vi "MovePilMotToRef.vi"(6 "Type de mouvement":T1 items=["Mouvement Simple"=1, "Aller vers Cote"=2], 7 "Variables d'Axes":T2={"OrdreBloc"="ni.var.psp://localhost/OPC/OPC1/esbimETH_1/module1/2AXBOC/E0_Ordre/Axe1_OrdreBloc", "Ordre UC"="ni.var.psp://localhost/OPC/OPC1/esbimETH_1/module1/2AXBOC/E0_Ordre/Axe1_OrdreUC", "CoteAAtteindre"="ni.var.psp://localhost/OPC/OPC1/esbimETH_1/module1/2AXBOC/E1_Position1/CoteAAtteindre", "Vitesse"="ni.var.psp://localhost/OPC/OPC1/esbimETH_1/module1/2AXBOC/E1_Position1/Vitesse", "Position codeur en pas"="ni.var.psp://localhost/OPC/OPC1/esbimETH_1/module1/2AXBOC/L4_PositionPas/Axe1_PositionCodeurEnPas", "Position Théorique"="ni.var.psp://localhost/OPC/OPC1/esbimETH_1/module1/2AXBOC/L0_Position/Axe1_PositionTheorique", "Message"="ni.var.psp://localhost/OPC/OPC1/esbimETH_1/module1/2AXBOC/L0_Position/Axe1_Messages", "Ecrire"="ni.var.psp://localhost/OPC/OPC1/esbimETH_1/module1/2AXBOC/ecrire", "Zone à écrire"="ni.var.psp://localhost/OPC/OPC1/esbimETH_1/module1/2AXBOC/zones_a_ecrire"}, 8 "error in (no error)":errorcluster caption="entrée d'erreur (pas d'erreur)", 9 "Vitesse":i32, 10 "Cote à atteindre":i32, 11 "Ordre UC":u16=1) -> (0 "error out":errorcluster caption="sortie d'erreur")   [LabVIEW 2012]
uses:
  Commandes/Type de Mouvement PilMOT.ctl
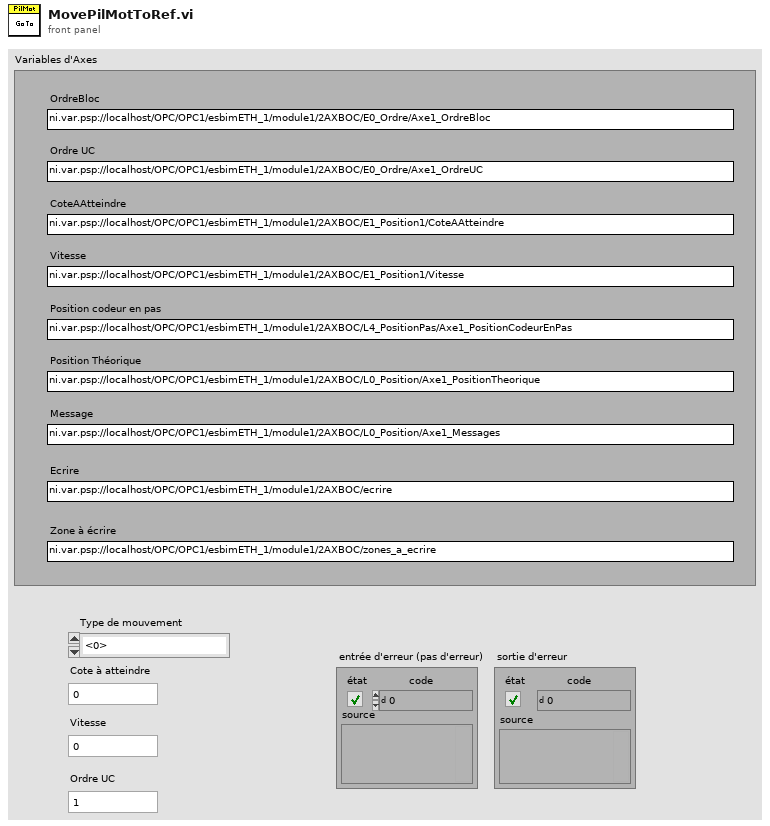
[diagram p1: front panel]
types:
  T1 = typedef "Type de Mouvement PilMOT.ctl" = u16
  T2 = cluster{"OrdreBloc":string, "Ordre UC":string, "CoteAAtteindre":string, "Vitesse":string, "Position codeur en pas":string, "Position Théorique":string, "Message":string, "Ecrire":string, "Zone à écrire":string}
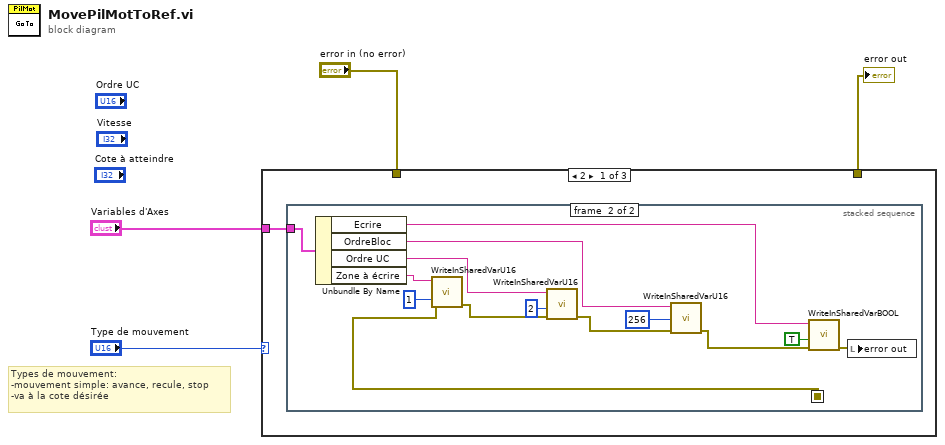
[diagram p0: block diagram]
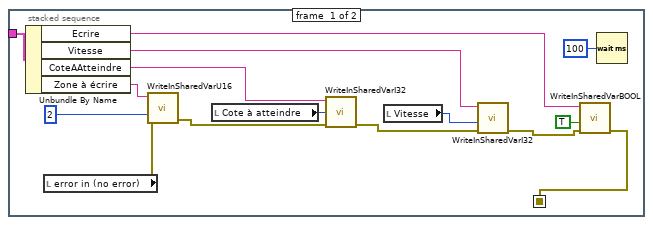
[diagram p2: hidden frame]
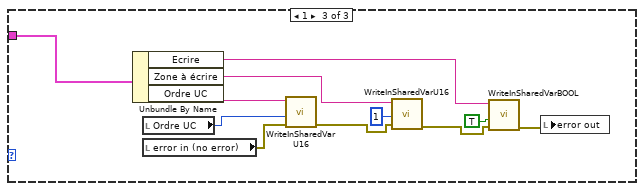
[diagram p4: hidden frame]
diagram:
  # "Types de mouvement:\n-mouvement simple: avance, recule, stop\n-va à la cote désirée"
  n1 = case shown="2" "Type de mouvement" {
    tunnel: "Variables d'Axes" -> [w5 _ w46]
    tunnel: [_ w35 _] -> w4
    tunnel: "error in (no error)" -> [_ w35 _]
    frame 2 {
      n2 = stacked-sequence {
        seq-local: [w10 _] -> [_ w33]
        tunnel: w5 -> [w20 w34]
        frame #0 {
          n3 = Unbundle By Name(w20) -> ("Ecrire"=w11:string, "Vitesse"=w15:string, "CoteAAtteindre"=w16:string, "Zone à écrire"=w18:string)
          n4 = local read "error in (no error)"() -> (w19:errorcluster)
          n5 = call "WriteInSharedVarU16.vi"("entrée d'erreur (pas d'erreur)"=w19, "données en entrée"=u16 2, "refnum de variable partagée en entrée"=w18) -> ("sortie d'erreur"=w17:errorcluster)  [unwired: 8 in]
          n6 = local read "Cote à atteindre"() -> (w9:i32)
          n7 = call "WriteInSharedVarI32.vi"("entrée d'erreur (pas d'erreur)"=w17, "données en entrée"=w9, "refnum de variable partagée en entrée"=w16) -> ("sortie d'erreur"=w14:errorcluster)  [unwired: 8 in]
          n8 = local read "Vitesse"() -> (w7:i32)
          n9 = call "WriteInSharedVarI32.vi"("entrée d'erreur (pas d'erreur)"=w14, "données en entrée"=w7, "refnum de variable partagée en entrée"=w15) -> ("sortie d'erreur"=w12:errorcluster)  [unwired: 8 in]
          n10 = call "WriteInSharedVarBOOL.vi"("entrée d'erreur (pas d'erreur)"=w12, "données en entrée"=TRUE, "refnum de variable partagée en entrée"=w11) -> ("sortie d'erreur"=w10:errorcluster)  [unwired: 8 in]
          n11 = Wait (ms)(milliseconds to wait=u32 100 ("attente (ms)")) -> ()  [unwired: 1 out]
        }
        frame #1 {
          n12 = Unbundle By Name(w34) -> ("Ecrire"=w26:string, "OrdreBloc"=w27:string, "Ordre UC"=w28:string, "Zone à écrire"=w32:string)
          n13 = call "WriteInSharedVarU16.vi"("entrée d'erreur (pas d'erreur)"=w33, "données en entrée"=u16 1, "refnum de variable partagée en entrée"=w32) -> ("sortie d'erreur"=w31:errorcluster)  [unwired: 8 in]
          n14 = call "WriteInSharedVarU16.vi"("entrée d'erreur (pas d'erreur)"=w31, "données en entrée"=u16 2, "refnum de variable partagée en entrée"=w28) -> ("sortie d'erreur"=w29:errorcluster)  [unwired: 8 in]
          n15 = call "WriteInSharedVarU16.vi"("entrée d'erreur (pas d'erreur)"=w29, "données en entrée"=u16 256, "refnum de variable partagée en entrée"=w27) -> ("sortie d'erreur"=w30:errorcluster)  [unwired: 8 in]
          n16 = call "WriteInSharedVarBOOL.vi"("entrée d'erreur (pas d'erreur)"=w30, "données en entrée"=TRUE, "refnum de variable partagée en entrée"=w26) -> ("sortie d'erreur"=w24:errorcluster)  [unwired: 8 in]
          n17 = local write "error out"(w24) -> ()
        }
      }
    }
    frame 0, Default {
    }
    frame 1 {
      n18 = Unbundle By Name(w46) -> ("Ecrire"=w40:string, "Zone à écrire"=w42:string, "Ordre UC"=w45:string)
      n19 = local read "Ordre UC"() -> (w37:u16)
      n20 = local read "error in (no error)"() -> (w44:errorcluster)
      n21 = call "WriteInSharedVarU16.vi"("entrée d'erreur (pas d'erreur)"=w44, "données en entrée"=w37, "refnum de variable partagée en entrée"=w45) -> ("sortie d'erreur"=w43:errorcluster)  [unwired: 8 in]
      n22 = call "WriteInSharedVarU16.vi"("entrée d'erreur (pas d'erreur)"=w43, "données en entrée"=u16 1, "refnum de variable partagée en entrée"=w42) -> ("sortie d'erreur"=w39:errorcluster)  [unwired: 8 in]
      n23 = call "WriteInSharedVarBOOL.vi"("entrée d'erreur (pas d'erreur)"=w39, "données en entrée"=TRUE, "refnum de variable partagée en entrée"=w40) -> ("sortie d'erreur"=w38:errorcluster)  [unwired: 8 in]
      n24 = local write "error out"(w38) -> ()
    }
  }
  "error out" <- w4
